vi "WPI_CAN_PCMGlobal.vi"(6 "Set Value":bool, 7 "Write After Receive":T2, 8 "Solenoid Set Mask":u8, 9 "Solenoid Set Value":u8, 10 "Operation":T4, 11 "Pneumatics Control Module (0)":u8) -> (1 "Get All":T1, 3 "Pneumatics Control Module Out":u8, 5 "Read For Send":T3={"Solenoids"=[FALSE, FALSE, FALSE, FALSE, FALSE, FALSE, FALSE, FALSE], "Closed Loop Enable"=FALSE, "Clear Sticky Faults"=FALSE, "Control Frame Rate Ms"=20})   [LabVIEW 2017]
uses:
  <vilib>/Rock Robotics/WPI/CAN/PCM/WPI_CAN_PCMGlobalOps.ctl
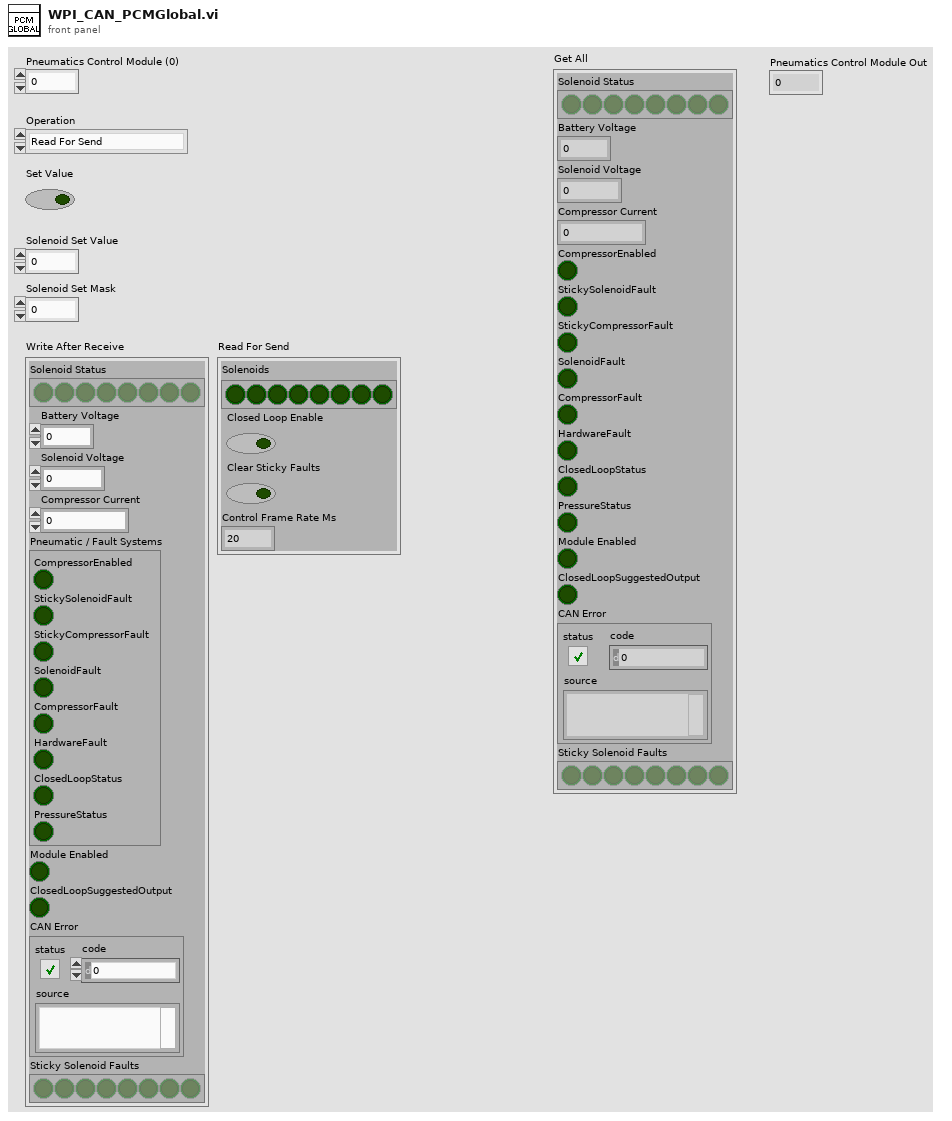
[diagram p1: front panel]
types:
  T1 = cluster{"Solenoid Status":bool[], "Battery Voltage":dbl, "Solenoid Voltage":dbl, "Compressor Current":dbl, "CompressorEnabled":bool, "StickySolenoidFault":bool, "StickyCompressorFault":bool, "SolenoidFault":bool, "CompressorFault":bool, "HardwareFault":bool, "ClosedLoopStatus":bool, "PressureStatus":bool, "Module Enabled":bool, "ClosedLoopSuggestedOutput":bool, "CAN Error":errorcluster, "Sticky Solenoid Faults":bool[]}
  T2 = cluster{"Solenoid Status":bool[], "Battery Voltage":dbl, "Solenoid Voltage":dbl, "Compressor Current":dbl, "Pneumatic / Fault Systems":cluster{"CompressorEnabled":bool, "StickySolenoidFault":bool, "StickyCompressorFault":bool, "SolenoidFault":bool, "CompressorFault":bool, "HardwareFault":bool, "ClosedLoopStatus":bool, "PressureStatus":bool}, "Module Enabled":bool, "ClosedLoopSuggestedOutput":bool, "CAN Error":errorcluster, "Sticky Solenoid Faults":bool[]}
  T3 = cluster{"Solenoids":bool[], "Closed Loop Enable":bool, "Clear Sticky Faults":bool, "Control Frame Rate Ms":i32}
  T4 = typedef "WPI_CAN_PCMGlobalOps.ctl" = enum16{"Read For Send", "Write After Receive", "Set Solenoids", "Set Closed Loop", "Clear Sticky Faults", "Get All", "Write Error", "Write After Receive Blacklist", "Set Control Frame Rate"}
  T5 = cluster{"Solenoids":bool[], "Closed Loop Enable":bool, "Clear Sticky Faults":bool, "Control Frame Rate Ms":i32}[]
  T6 = cluster{"Solenoid Status":bool[], "Battery Voltage":dbl, "Solenoid Voltage":dbl, "Compressor Current":dbl, "Status":cluster{"CompressorEnabled":bool, "StickySolenoidFault":bool, "StickyCompressorFault":bool, "SolenoidFault":bool, "CompressorFault":bool, "HardwareFault":bool, "ClosedLoopStatus":bool, "PressureStatus":bool}, "Module Enabled":bool, "ClosedLoopSuggestedOutput":bool, "CAN Error":errorcluster, "Sticky Solenoid Faults":bool[]}[]
  T7 = cluster{"Solenoid Status":bool[], "Battery Voltage":dbl, "Solenoid Voltage":dbl, "Compressor Current":dbl, "Status":cluster{"CompressorEnabled":bool, "StickySolenoidFault":bool, "StickyCompressorFault":bool, "SolenoidFault":bool, "CompressorFault":bool, "HardwareFault":bool, "ClosedLoopStatus":bool, "PressureStatus":bool}, "Module Enabled":bool, "ClosedLoopSuggestedOutput":bool, "CAN Error":errorcluster, "Sticky Solenoid Faults":bool[]}
  T8 = cluster{"CompressorEnabled":bool, "StickySolenoidFault":bool, "StickyCompressorFault":bool, "SolenoidFault":bool, "CompressorFault":bool, "HardwareFault":bool, "ClosedLoopStatus":bool, "PressureStatus":bool}
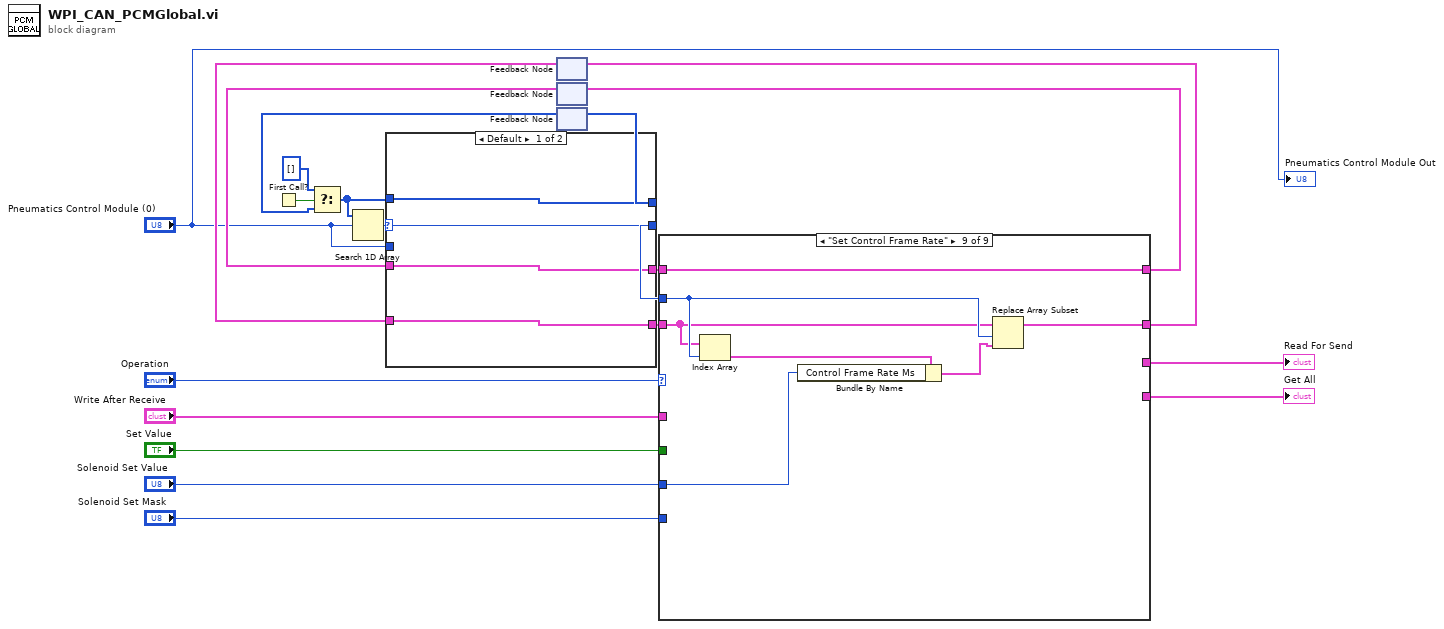
[diagram p0: block diagram]
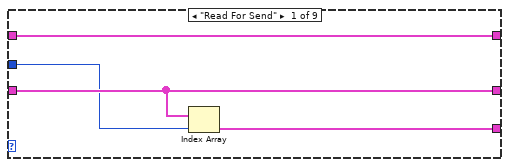
[diagram p2: hidden frame]
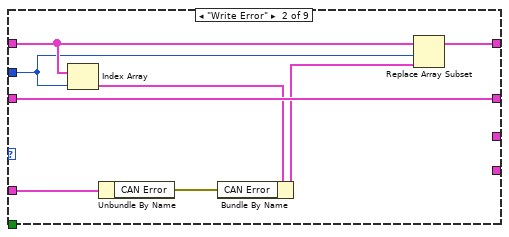
[diagram p3: hidden frame]
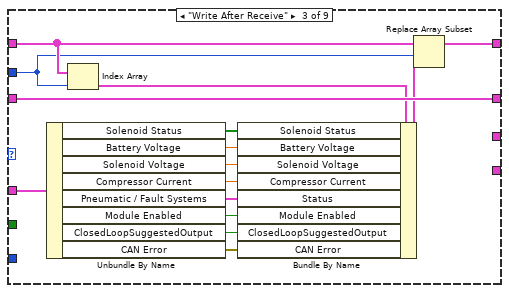
[diagram p4: hidden frame]
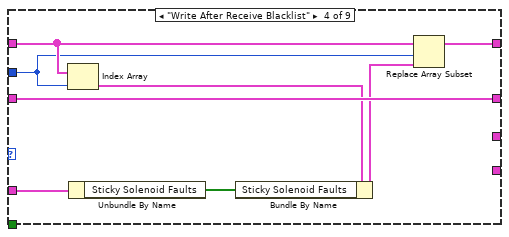
[diagram p5: hidden frame]
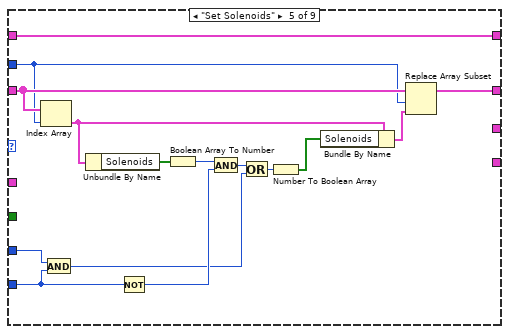
[diagram p6: hidden frame]
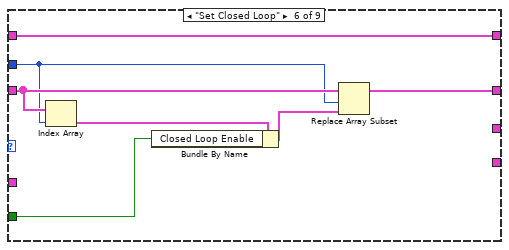
[diagram p7: hidden frame]
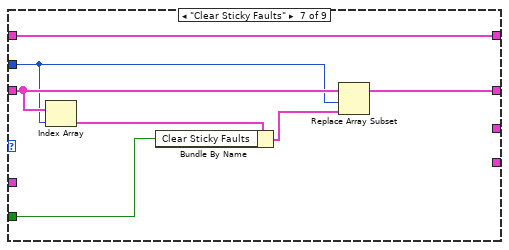
[diagram p8: hidden frame]
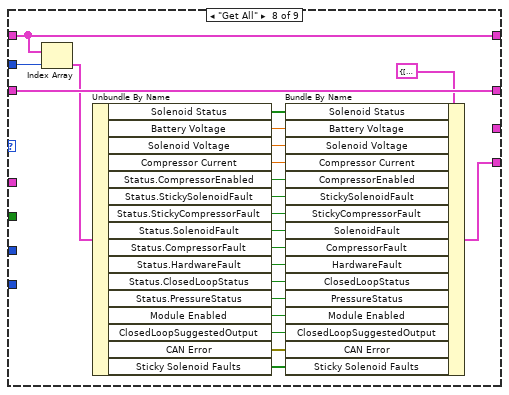
[diagram p9: hidden frame]
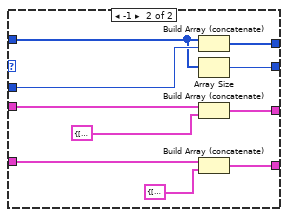
[diagram p10: hidden frame]
diagram:
  n1 = First Call?() -> (First Call?: T/F=w21:bool)
  n2 = feedback #1() -> (w14:T5)  [unwired: 1 in]
  n3 = feedback #2() -> (w15:T6)  [unwired: 1 in]
  n4 = feedback #3() -> (w19:u8[])  [unwired: 1 in]
  n5 = Select(t=u8[] [], s=w21, f=w19) -> (s? t:f=w17:u8[])
  n6 = Search 1D Array(1D array=w17, element="Pneumatics Control Module (0)") -> (index of element=w16:i32)  [unwired: 1 in]
  n7 = case shown="Default" w16 {
    selector: w16 -> [w22 _]
    tunnel: [w25 w35] -> w18
    tunnel: "Pneumatics Control Module (0)" -> [_ w34]
    tunnel: w17 -> [w25 w28]
    tunnel: w15 -> [w24 w33]
    tunnel: w14 -> [w23 w31]
    tunnel: [w24 w30] -> w12
    tunnel: [w23 w29] -> w10
    tunnel: [w22 w27] -> w8
    frame Default {
    }
    frame -1 {
      n8 = Build Array (concatenate)(w28, w34) -> (w35:u8[])
      n9 = Array Size(array=w28) -> (size(s)=w27:i32)
      n10 = Build Array (concatenate)(w33, T7 {"Solenoid Status"=[FALSE, FALSE, FALSE, FALSE, FALSE, FALSE, FALSE, FALSE], "Battery Voltage"=0.0, "Solenoid Voltage"=0.0, "Compressor Current"=0.0, "Status"={"CompressorEnabled"=FALSE, "StickySolenoidFault"=FALSE, "StickyCompressorFault"=FALSE, "SolenoidFault"=FALSE, "CompressorFault"=FALSE, "HardwareFault"=FALSE, "ClosedLoopStatus"=FALSE, "PressureStatus"=FALSE}, "Module Enabled"=FALSE, "ClosedLoopSuggestedOutput"=FALSE, "CAN Error"={"status"=FALSE, "code"=0, "source"=""}, "Sticky Solenoid Faults"=[FALSE, FALSE, FALSE, FALSE, FALSE, FALSE, FALSE, FALSE]} ("Write After Receive")) -> (w30:T6)
      n11 = Build Array (concatenate)(w31, T3 {"Solenoids"=[FALSE, FALSE, FALSE, FALSE, FALSE, FALSE, FALSE, FALSE], "Closed Loop Enable"=FALSE, "Clear Sticky Faults"=FALSE, "Control Frame Rate Ms"=20} ("Read For Send")) -> (w29:T5)
    }
  }
  n12 = feedback-in #3(w18) -> ()
  n13 = case shown="\"Set Control Frame Rate\"" "Operation" {
    tunnel: [w39 w46 w61 w69 w85 w86 w93 w119 w128] -> w13
    tunnel: w12 -> [w39 w45 w60 w68 w85 w86 w93 w119 w128]
    tunnel: [w38 w47 w62 w70 w83 w92 w99 w121 w127] -> w11
    tunnel: w10 -> [w38 w47 w62 w70 w84 w91 w98 w121 w124]
    tunnel: w8 -> [w37 w44 w59 w67 w82 w90 w97 w120 w126]
    tunnel: [w36 _ _ _ _ _ _ _ _] -> w7
    tunnel: "Write After Receive" -> [_ w41 w56 w64 _ _ _ _ _]
    tunnel: "Solenoid Set Value" -> [_ _ _ _ w80 _ _ _ w123]
    tunnel: "Solenoid Set Mask" -> [_ _ _ _ w79 _ _ _ _]
    tunnel: "Set Value" -> [_ _ _ _ _ w87 w94 _ _]
    tunnel: [_ _ _ _ _ _ _ w117 _] -> w2
    frame "Read For Send" {
      n14 = Index Array(array=w38, index=w37) -> (element=w36:T3)
    }
    frame "Write Error" {
      n15 = Index Array(array=w45, index=w44) -> (element=w43:T7)
      n16 = Unbundle By Name(w41) -> ("CAN Error"=w40:errorcluster)
      n17 = Bundle By Name(cluster=w43, "CAN Error"=w40) -> (w42:T7)
      n18 = Replace Array Subset(array=w45, new element=w42, index=w44) -> (w46:T6)
    }
    frame "Write After Receive" {
      n19 = Unbundle By Name(w56) -> ("Solenoid Status"=w55:bool[], "Battery Voltage"=w54:dbl, "Solenoid Voltage"=w53:dbl, "Compressor Current"=w52:dbl, "Pneumatic / Fault Systems"=w51:T8, "Module Enabled"=w50:bool, "ClosedLoopSuggestedOutput"=w49:bool, "CAN Error"=w48:errorcluster)
      n20 = Index Array(array=w60, index=w59) -> (element=w58:T7)
      n21 = Bundle By Name(cluster=w58, "Solenoid Status"=w55, "Battery Voltage"=w54, "Solenoid Voltage"=w53, "Compressor Current"=w52, "Status"=w51, "Module Enabled"=w50, "ClosedLoopSuggestedOutput"=w49, "CAN Error"=w48) -> (w57:T7)
      n22 = Replace Array Subset(array=w60, new element=w57, index=w59) -> (w61:T6)
    }
    frame "Write After Receive Blacklist" {
      n23 = Index Array(array=w68, index=w67) -> (element=w66:T7)
      n24 = Unbundle By Name(w64) -> ("Sticky Solenoid Faults"=w63:bool[])
      n25 = Bundle By Name(cluster=w66, "Sticky Solenoid Faults"=w63) -> (w65:T7)
      n26 = Replace Array Subset(array=w68, new element=w65, index=w67) -> (w69:T6)
    }
    frame "Set Solenoids" {
      n27 = Index Array(array=w84, index=w82) -> (element=w74:T3)
      n28 = And(x=w80, y=w79) -> (x .and. y?=w75:u8)
      n29 = Unbundle By Name(w74) -> ("Solenoids"=w81:bool[])
      n30 = Not(x=w79) -> (.not. x?=w77:u8)
      n31 = Boolean Array To Number(Boolean array=w81) -> (number=w78:u8)
      n32 = And(x=w78, y=w77) -> (x .and. y?=w76:u8)
      n33 = Or(x=w76, y=w75) -> (x .or. y?=w73:u8)
      n34 = Number To Boolean Array(number=w73) -> (Boolean array=w72:bool[])
      n35 = Bundle By Name(cluster=w74, "Solenoids"=w72) -> (w71:T3)
      n36 = Replace Array Subset(array=w84, new element=w71, index=w82) -> (w83:T5)
    }
    frame "Set Closed Loop" {
      n37 = Index Array(array=w91, index=w90) -> (element=w89:T3)
      n38 = Bundle By Name(cluster=w89, "Closed Loop Enable"=w87) -> (w88:T3)
      n39 = Replace Array Subset(array=w91, new element=w88, index=w90) -> (w92:T5)
    }
    frame "Clear Sticky Faults" {
      n40 = Index Array(array=w98, index=w97) -> (element=w96:T3)
      n41 = Bundle By Name(cluster=w96, "Clear Sticky Faults"=w94) -> (w95:T3)
      n42 = Replace Array Subset(array=w98, new element=w95, index=w97) -> (w99:T5)
    }
    frame "Get All" {
      n43 = Index Array(array=w119, index=w120) -> (element=w118:T7)
      n44 = Unbundle By Name(w118) -> ("Solenoid Status"=w116:bool[], "Battery Voltage"=w115:dbl, "Solenoid Voltage"=w114:dbl, "Compressor Current"=w113:dbl, "Status.CompressorEnabled"=w112:bool, "Status.StickySolenoidFault"=w111:bool, "Status.StickyCompressorFault"=w110:bool, "Status.SolenoidFault"=w109:bool, "Status.CompressorFault"=w108:bool, "Status.HardwareFault"=w107:bool, "Status.ClosedLoopStatus"=w106:bool, "Status.PressureStatus"=w105:bool, "Module Enabled"=w104:bool, "ClosedLoopSuggestedOutput"=w103:bool, "CAN Error"=w102:errorcluster, "Sticky Solenoid Faults"=w100:bool[])
      n45 = Bundle By Name(cluster=T1 {"Solenoid Status"=[], "Battery Voltage"=0.0, "Solenoid Voltage"=0.0, "Compressor Current"=0.0, "CompressorEnabled"=FALSE, "StickySolenoidFault"=FALSE, "StickyCompressorFault"=FALSE, "SolenoidFault"=FALSE, "CompressorFault"=FALSE, "HardwareFault"=FALSE, "ClosedLoopStatus"=FALSE, "PressureStatus"=FALSE, "Module Enabled"=FALSE, "ClosedLoopSuggestedOutput"=FALSE, "CAN Error"={"status"=FALSE, "code"=0, "source"=""}, "Sticky Solenoid Faults"=[]} ("Get All"), "Solenoid Status"=w116, "Battery Voltage"=w115, "Solenoid Voltage"=w114, "Compressor Current"=w113, "CompressorEnabled"=w112, "StickySolenoidFault"=w111, "StickyCompressorFault"=w110, "SolenoidFault"=w109, "CompressorFault"=w108, "HardwareFault"=w107, "ClosedLoopStatus"=w106, "PressureStatus"=w105, "Module Enabled"=w104, "ClosedLoopSuggestedOutput"=w103, "CAN Error"=w102, "Sticky Solenoid Faults"=w100) -> (w117:T1)
    }
    frame "Set Control Frame Rate" {
      n46 = Index Array(array=w124, index=w126) -> (element=w125:T3)
      n47 = Bundle By Name(cluster=w125, "Control Frame Rate Ms"=w123) -> (w122:T3)
      n48 = Replace Array Subset(array=w124, new element=w122, index=w126) -> (w127:T5)
    }
  }
  "Read For Send" <- w7
  "Get All" <- w2
  n49 = feedback-in #1(w11) -> ()
  n50 = feedback-in #2(w13) -> ()
  "Pneumatics Control Module Out" <- "Pneumatics Control Module (0)"
